vi "Cloud.vi"() -> ()   [LabVIEW 2017]
uses:
  <vilib>/daq.io/daq.io LabVIEW API/_typedefs/daqio-Credentials.ctl
  <vilib>/daq.io/daq.io LabVIEW API/_subs/daqio_Write_Single.vi
  <vilib>/daq.io/daq.io LabVIEW API/daqio minimal.lvlib
panel:
  in  "Stop Button":bool
  in  "Credentials":T1
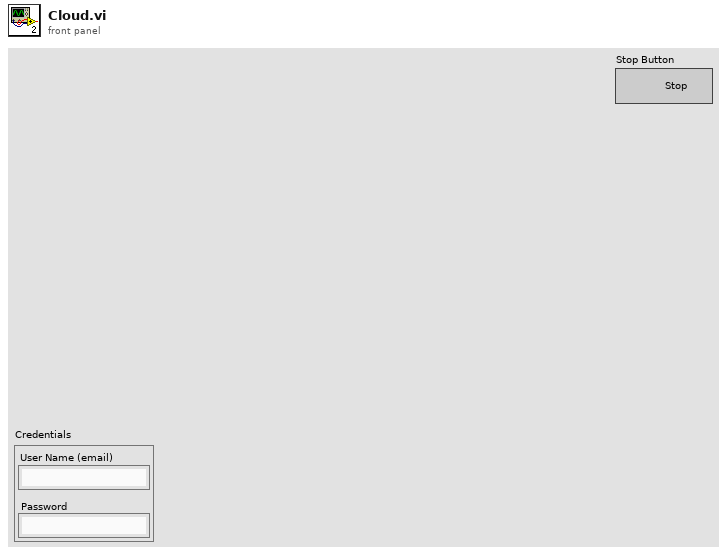
[diagram p1: front panel]
types:
  T1 = typedef "daqio minimal.lvlib/daqio-Credentials.ctl" = cluster{"User Name (email)":string, "Password":string}
  T2 = typedef "daqio minimal.lvlib/daqio-Type.ctl" = cluster{"daq.io ref":T3, "daq.io API Base":string, "Device Key":string, "Account ID":string, "online":bool, "SSL":bool, "buffer":bool}
  T3 = typedef "LabVIEWHTTPClient.lvlib/ClientHandle.ctl" = refnum<k1>
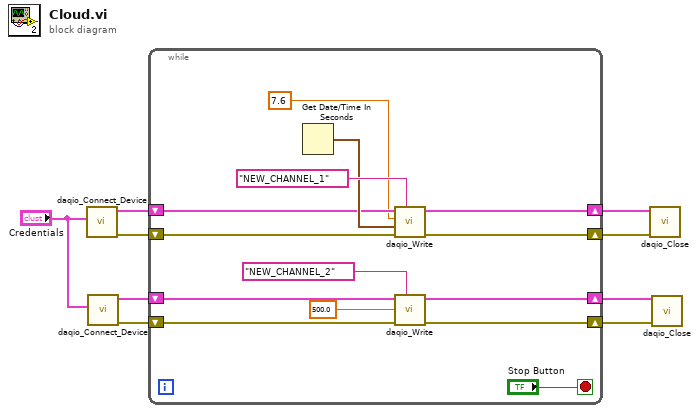
[diagram p0: block diagram]
diagram:
  n1 = call <vilib>:"daqio_Connect_Device.vi"("Credentials"="Credentials") -> ("error out"=w8:errorcluster, "daq.io type out"=w9:T2)  [unwired: 8 in, 1 out]
  n2 = call <vilib>:"daqio_Connect_Device.vi"("Credentials"="Credentials") -> ("error out"=w4:errorcluster, "daq.io type out"=w5:T2)  [unwired: 8 in, 1 out]
  n3 = while {
    shift-right: [w19] -> w7
    shift-left: w9 -> [w21]
    shift-right: [w18] -> w6
    shift-left: w8 -> [w20]
    shift-right: [w14] -> w3
    shift-left: w5 -> [w16]
    shift-right: [w13] -> w2
    shift-left: w4 -> [w15]
    stop <- "Stop Button" stop-if-true
    n4 = Get Date/Time In Seconds() -> (seconds since 1Jan1904=w22:timestamp)
    n5 = call-poly <vilib>:"daqio_Write.vi"("daq.io Device Channel Key"="NEW_CHANNEL_1", "error in (no error)"=w20, "timestamp"=w22, "value"=7.6, "daq.io type in"=w21) -> ("error out"=w18:errorcluster, "daq.io type out"=w19:T2)  [unwired: 5 in]
    n6 = call-poly <vilib>:"daqio_Write.vi"("daq.io Device Channel Key"="NEW_CHANNEL_2", "error in (no error)"=w15, "value"=500.0, "daq.io type in"=w16) -> ("error out"=w13:errorcluster, "daq.io type out"=w14:T2)  [unwired: 6 in]
  }
  n7 = call <vilib>:"daqio_Close.vi"("error in (no error)"=w6, "daq.io type"=w7) -> ()  [unwired: 9 in, 1 out]
  n8 = call <vilib>:"daqio_Close.vi"("error in (no error)"=w2, "daq.io type"=w3) -> ()  [unwired: 9 in, 1 out]
